vi "Acquire Pulse Result.vi"(8 "error in (no error)":errorcluster, 11 "DAQmx Lockin Digitizer Driver in":refnum<class "DAQmx Lockin Digitizer Driver.lvclass">) -> (0 "error out":errorcluster, 2 "Pulse acquired":bool, 3 "DAQmx Lockin Digitizer Driver out":refnum<class "DAQmx Lockin Digitizer Driver.lvclass">)   [LabVIEW 2021, in "DAQmx Lockin Digitizer Driver.lvclass"]
uses:
  DAQmx Lockin Digitizer Driver.lvclass
  C:/GitHub/NHMFL_Core/Libraries/NI-DAQ/DAQmx Digitizer/DAQmx Digitizer.lvclass
  DAQmx Lockin Driver/DAQmx Lockin Driver.lvclass
  DAQmx Lockin Digitizer Driver.lvclass/DAQmx Lockin Digitizer Driver.ctl
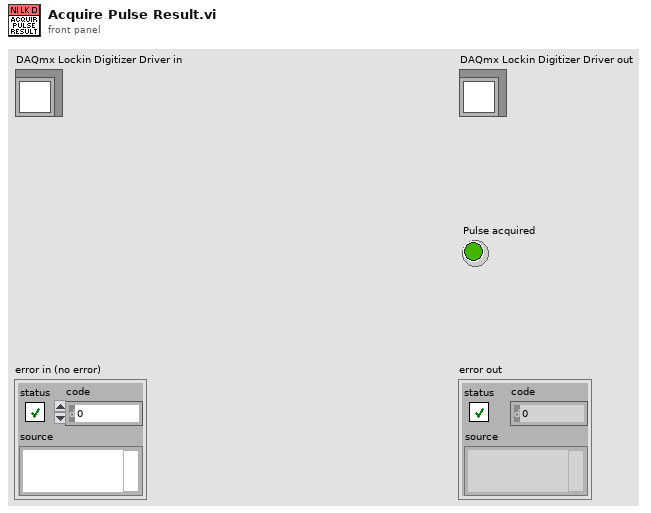
[diagram p1: front panel]
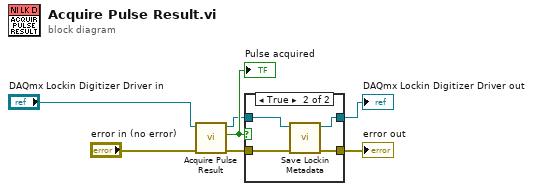
[diagram p0: block diagram]
diagram:
  n1 = call-parent "Acquire Pulse Result.vi"("error in (no error)"="error in (no error)", "Pulse Driver in"="DAQmx Lockin Digitizer Driver in") -> ("error out"=w3:errorcluster, "Pulse acquired"=w5:bool, "Pulse Driver out"=w4:refnum<class "DAQmx Lockin Digitizer Driver.lvclass">)  [unwired: 7 in]
  "Pulse acquired" <- w5
  n2 = case shown="True" w5 {
    tunnel: w4 -> [w8 w10]
    tunnel: w3 -> [w9 w13]
    tunnel: [w9 w12] -> w2
    tunnel: [w8 w11] -> w1
    frame False {
    }
    frame True {
      n3 = call-dynamic "Save Lockin Metadata.vi"("error in (no error)"=w13, "DAQmx Lockin Digitizer Driver in"=w10) -> ("error out"=w12:errorcluster, "DAQmx Lockin Digitizer Driver out"=w11:refnum<class "DAQmx Lockin Digitizer Driver.lvclass">)  [unwired: 8 in]
    }
  }
  "error out" <- w2
  "DAQmx Lockin Digitizer Driver out" <- w1
